vi "scaleFeaturesPositions_YZ_um_pix.vi"(8 "error in (no error)":errorcluster, 11 "?":T1={"PythonSession"=refnum, "Display"=FALSE, "BinThreshold"=0.0, "LIST HOLO BATCH"=[], "Display"=[], "meanHolo"=[], "FEATURES(µm)"=[], "LabelPicture"="", "Status"="", "planeToDisplayFeatures"=enum."XY", "State"=enum."WAIT"}) -> (0 "error out":errorcluster, 3 "XYFeatures(pix)":sgl[][](array[numeric]))   [LabVIEW 2023, in "holoPyTracks.lvlib"]
uses:
  HoloPyLib/holoPyTracks.lvlib
  datas.ctl
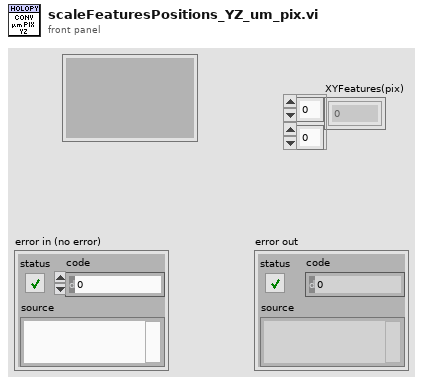
[diagram p1: front panel]
types:
  T1 = typedef "datas.ctl" = cluster{"PythonSession":refnum<k35>, "Display":bool, "BinThreshold":sgl, "LIST HOLO BATCH":path[], "Display":sgl[][], "meanHolo":sgl[][], "FEATURES(µm)":sgl[][], "LabelPicture":string, "Status":string, "planeToDisplayFeatures":enum16{"XY", "XZ", "YZ"}, "State":enum16{"SESSION CLOSED", "WAIT", "TEST WAIT", "TEST IN PROGESS", "BATCH IN PROGRESS"}}
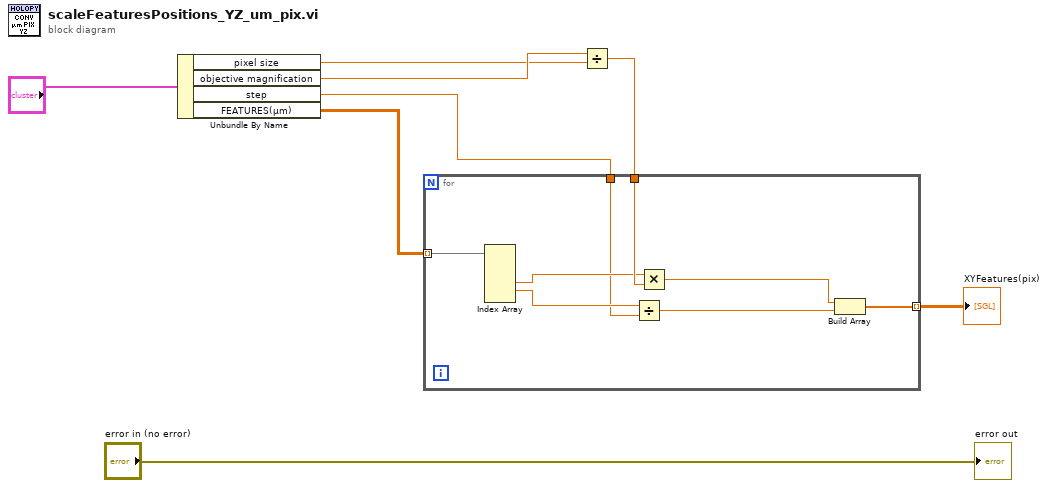
[diagram p0: block diagram]
diagram:
  n1 = Unbundle By Name("?") -> ("pixel size"=w7:sgl, "objective magnification"=w8:sgl, "step"=w1:dbl, "FEATURES(µm)"=w2:sgl[][])
  n2 = Divide(x=w8, y=w7) -> (x/y=w6:sgl)
  n3 = for {
    tunnel: w2 -> [w16] mode=indexing
    tunnel: w6 -> [w12]
    tunnel: [w14] -> w5 mode=indexing
    tunnel: w1 -> [w10]
    n4 = Index Array(array=w16) -> (element #3=w11:sgl, element #4=w13:sgl)  [unwired: 5 in, 3 out]
    n5 = Divide(x=w13, y=w10) -> (x/y=w9:dbl)
    n6 = Multiply(x=w11, y=w12) -> (x*y=w15:sgl)
    n7 = Build Array(w15, w9) -> (w14:dbl[])
  }
  "XYFeatures(pix)" <- w5
  "error out" <- "error in (no error)"
